vi "Add Class to Page Map.vi"(8 "error in (no error)":errorcluster {"code" format="Error %.0f"}, 9 "Class Qualified Name":string, 10 "Page Name":string, 11 "VIDoc Printer - Confluence In":refnum<class "VIDoc Printer - Confluence.lvclass">) -> (0 "error out":errorcluster {"code" format="Error %.0f"}, 3 "VIDoc Printer - Confluence Out":refnum<class "VIDoc Printer - Confluence.lvclass">)   [LabVIEW 2023, in "VIDoc Printer - Confluence.lvlib" / "VIDoc Printer - Confluence.lvclass"]
uses:
  VIDoc Printer - Confluence.lvclass
  VIDoc Printer - Confluence.lvclass/VIDoc Printer - Confluence.ctl
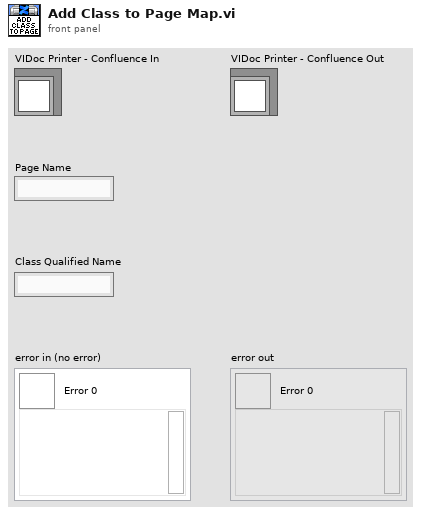
[diagram p1: front panel]
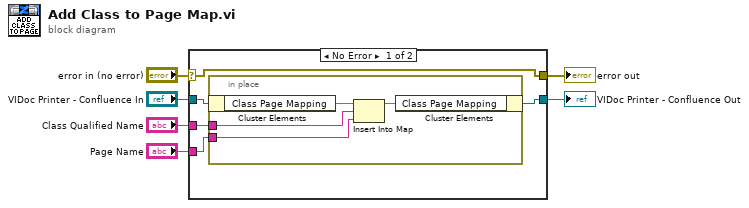
[diagram p0: block diagram]
diagram:
  n1 = case shown="No Error" "error in (no error)" {
    selector: "error in (no error)" -> [w11 w17]
    tunnel: [w11 w17] -> w5
    tunnel: [w9 w16] -> w3
    tunnel: "VIDoc Printer - Confluence In" -> [w10 w16]
    tunnel: "Class Qualified Name" -> [w8 _]
    tunnel: "Page Name" -> [w7 _]
    frame No Error {
      n2 = in-place {
        in-place-border: w8 -> [w13]
        in-place-border: w7 -> [w12]
        n3 = in-place-cluster #1(w10) -> ("Class Page Mapping"=w15:map{string, string})
        n4 = Insert Into Map(map in=w15, key=w13, value=w12) -> (map out=w14:map{string, string})  [unwired: 2 out]
        n5 = in-place-cluster #1("Class Page Mapping"=w14) -> (w9:refnum<class "VIDoc Printer - Confluence.lvclass">)
      }
    }
    frame Error {
    }
  }
  "error out" <- w5
  "VIDoc Printer - Confluence Out" <- w3
